vi "DriveStraight.vi"(6 "Reset":bool, 11 "Angle":dbl) -> (3 "Turn":dbl)   [LabVIEW 2016]
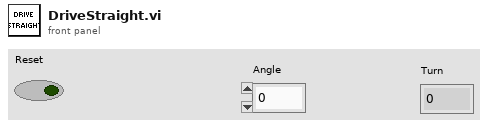
[diagram p1: front panel]
types:
  T1 = cluster{"proportional gain (Kc)":dbl, "integral time (Ti, min)":dbl, "derivative time (Td, min)":dbl}
  T2 = cluster{"Yaw":dbl, "Roll":dbl, "Pitch":dbl, "Heading":dbl, "Fused Heading":dbl}
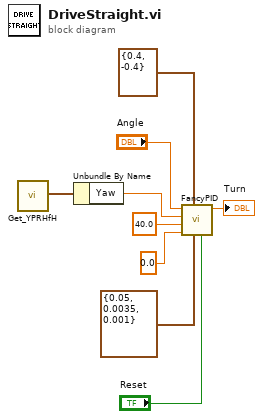
[diagram p0: block diagram]
diagram:
  n1 = call <vilib>:"Get_YPRHfH.vi"() -> ("YRPHfH"=w2:T2)  [unwired: 11 in]
  n2 = Unbundle By Name(w2) -> ("Yaw"=w1:dbl)
  n3 = call "FancyPID.vi"("Reset"="Reset", "Gains"=T1 {"proportional gain (Kc)"=0.05, "integral time (Ti, min)"=0.0035, "derivative time (Td, min)"=0.001}, "Range"=cluster{"output high":dbl, "output low":dbl} {"output high"=0.4, "output low"=-0.4}, "Disable Range"=0.0, "Integral Range"=40.0, "Process variable"=w1, "Setpoint"="Angle") -> ("output"=→"Turn":dbl)  [unwired: 4 in]
